vi "main.vi"() -> ()   [LabVIEW 2016]
uses:
  <vilib>/Utility/miscctls.llb/LVPointTypeDef.ctl
  <vilib>/Averna/Notify Icon/NotifyIcon.llb/BalloonIcon.ctl
  <vilib>/Averna/Notify Icon/NotifyIcon.llb/NotifyIcon.lvclass
  <vilib>/Utility/config.llb/NI_LVConfig.lvlib
  <vilib>/Utility/config.llb/Read Key (String).vi
  <vilib>/Utility/config.llb/Write Key (String).vi
  <vilib>/Utility/config.llb/Read Key (U32).vi
panel:
  in  "table元素":string
  in  "结果 2":bool
  out "数值":i32
  out "错误输出":errorcluster
  in  "连接ID":refnum<k5>
  out "结果":bool
  out "数组 2":string[](array[string])
  out "数据":string
  out "拆分包及应答Flag":string
  out "设备编码MN":string
  out "密码PW":string
  out "命令编码CN":string
  out "系统编码ST":string
  out "数组":string[](array[string])
  in  "站点名称":string(combo)
  out "时间标识":timestamp format="%<%Y/%m/%d %H:%M:%S>T"
  out "心跳包":bool
  out "空闲时间":dbl
  out "步骤":T1(ring)
  out "元素":string
  out "try":dbl
  in  "PW":string
  in  "MN":string
  in  "Port":u16
  in  "IP":string
  in  "停止 2":bool
  out "1st Error to Convert":i32(ring)=56 items=["无错误", "参数错误", "内存已满", "超出区域", "文件结束", "文件已打开", "一般文件IO错误", "未找到文件", "文件权限错误", "磁盘已满", "路径副本", "打开过多文件", "未启用", "未找到资源文件", "无法添加资源", "未找到资源", "未找到图像", "图像内存错误", "画笔不存在", "配置错误类型", "配置未找到解析段", "配置解析错误", "配置内存错误", "错误外部代码格式", "错误外部代码偏移量", "外部代码不存在", "空窗口", "销毁窗口错误", "空菜单", "打印已中止", "错误打印记录", "打印驱动程序错误", "打印时窗口错误", "打印时内存错误", "打印对话框错误", "一般打印错误", "无效设备引用句柄", "设备未找到", "设备参数错误", "设备单位错误", "无法打开设备", "设备调用已中止", "一般错误", "用户已取消", "对象ID过低", "对象ID过高", "对象不在堆中", "未知的堆", "错误DefProc ID", "DefProc不在表格中", "范围外信息", "空方法", "未知信息", "不支持管理器调用", "错误地址", "连接过程中", "连接超时", "连接过程中", "不支持网络属性", "网络错误", "正在使用的地址", "系统缺少内存", "连接已中止", "连接已拒绝", "连接未建立", "连接已建立", "连接已关闭", "初始化错误（交互应用程序管理器）", "错误事件发生", "等待无约束事件发生处理程序", "事件发生队列溢出", "错误路径", "未发出信号量", "未识别类型（交互应用程序管理器）"]
  out "读取上位机数据":string
  out "通讯包字符串":string
  out "字符串":string
  out "error out":errorcluster
  # "平台发送系统"
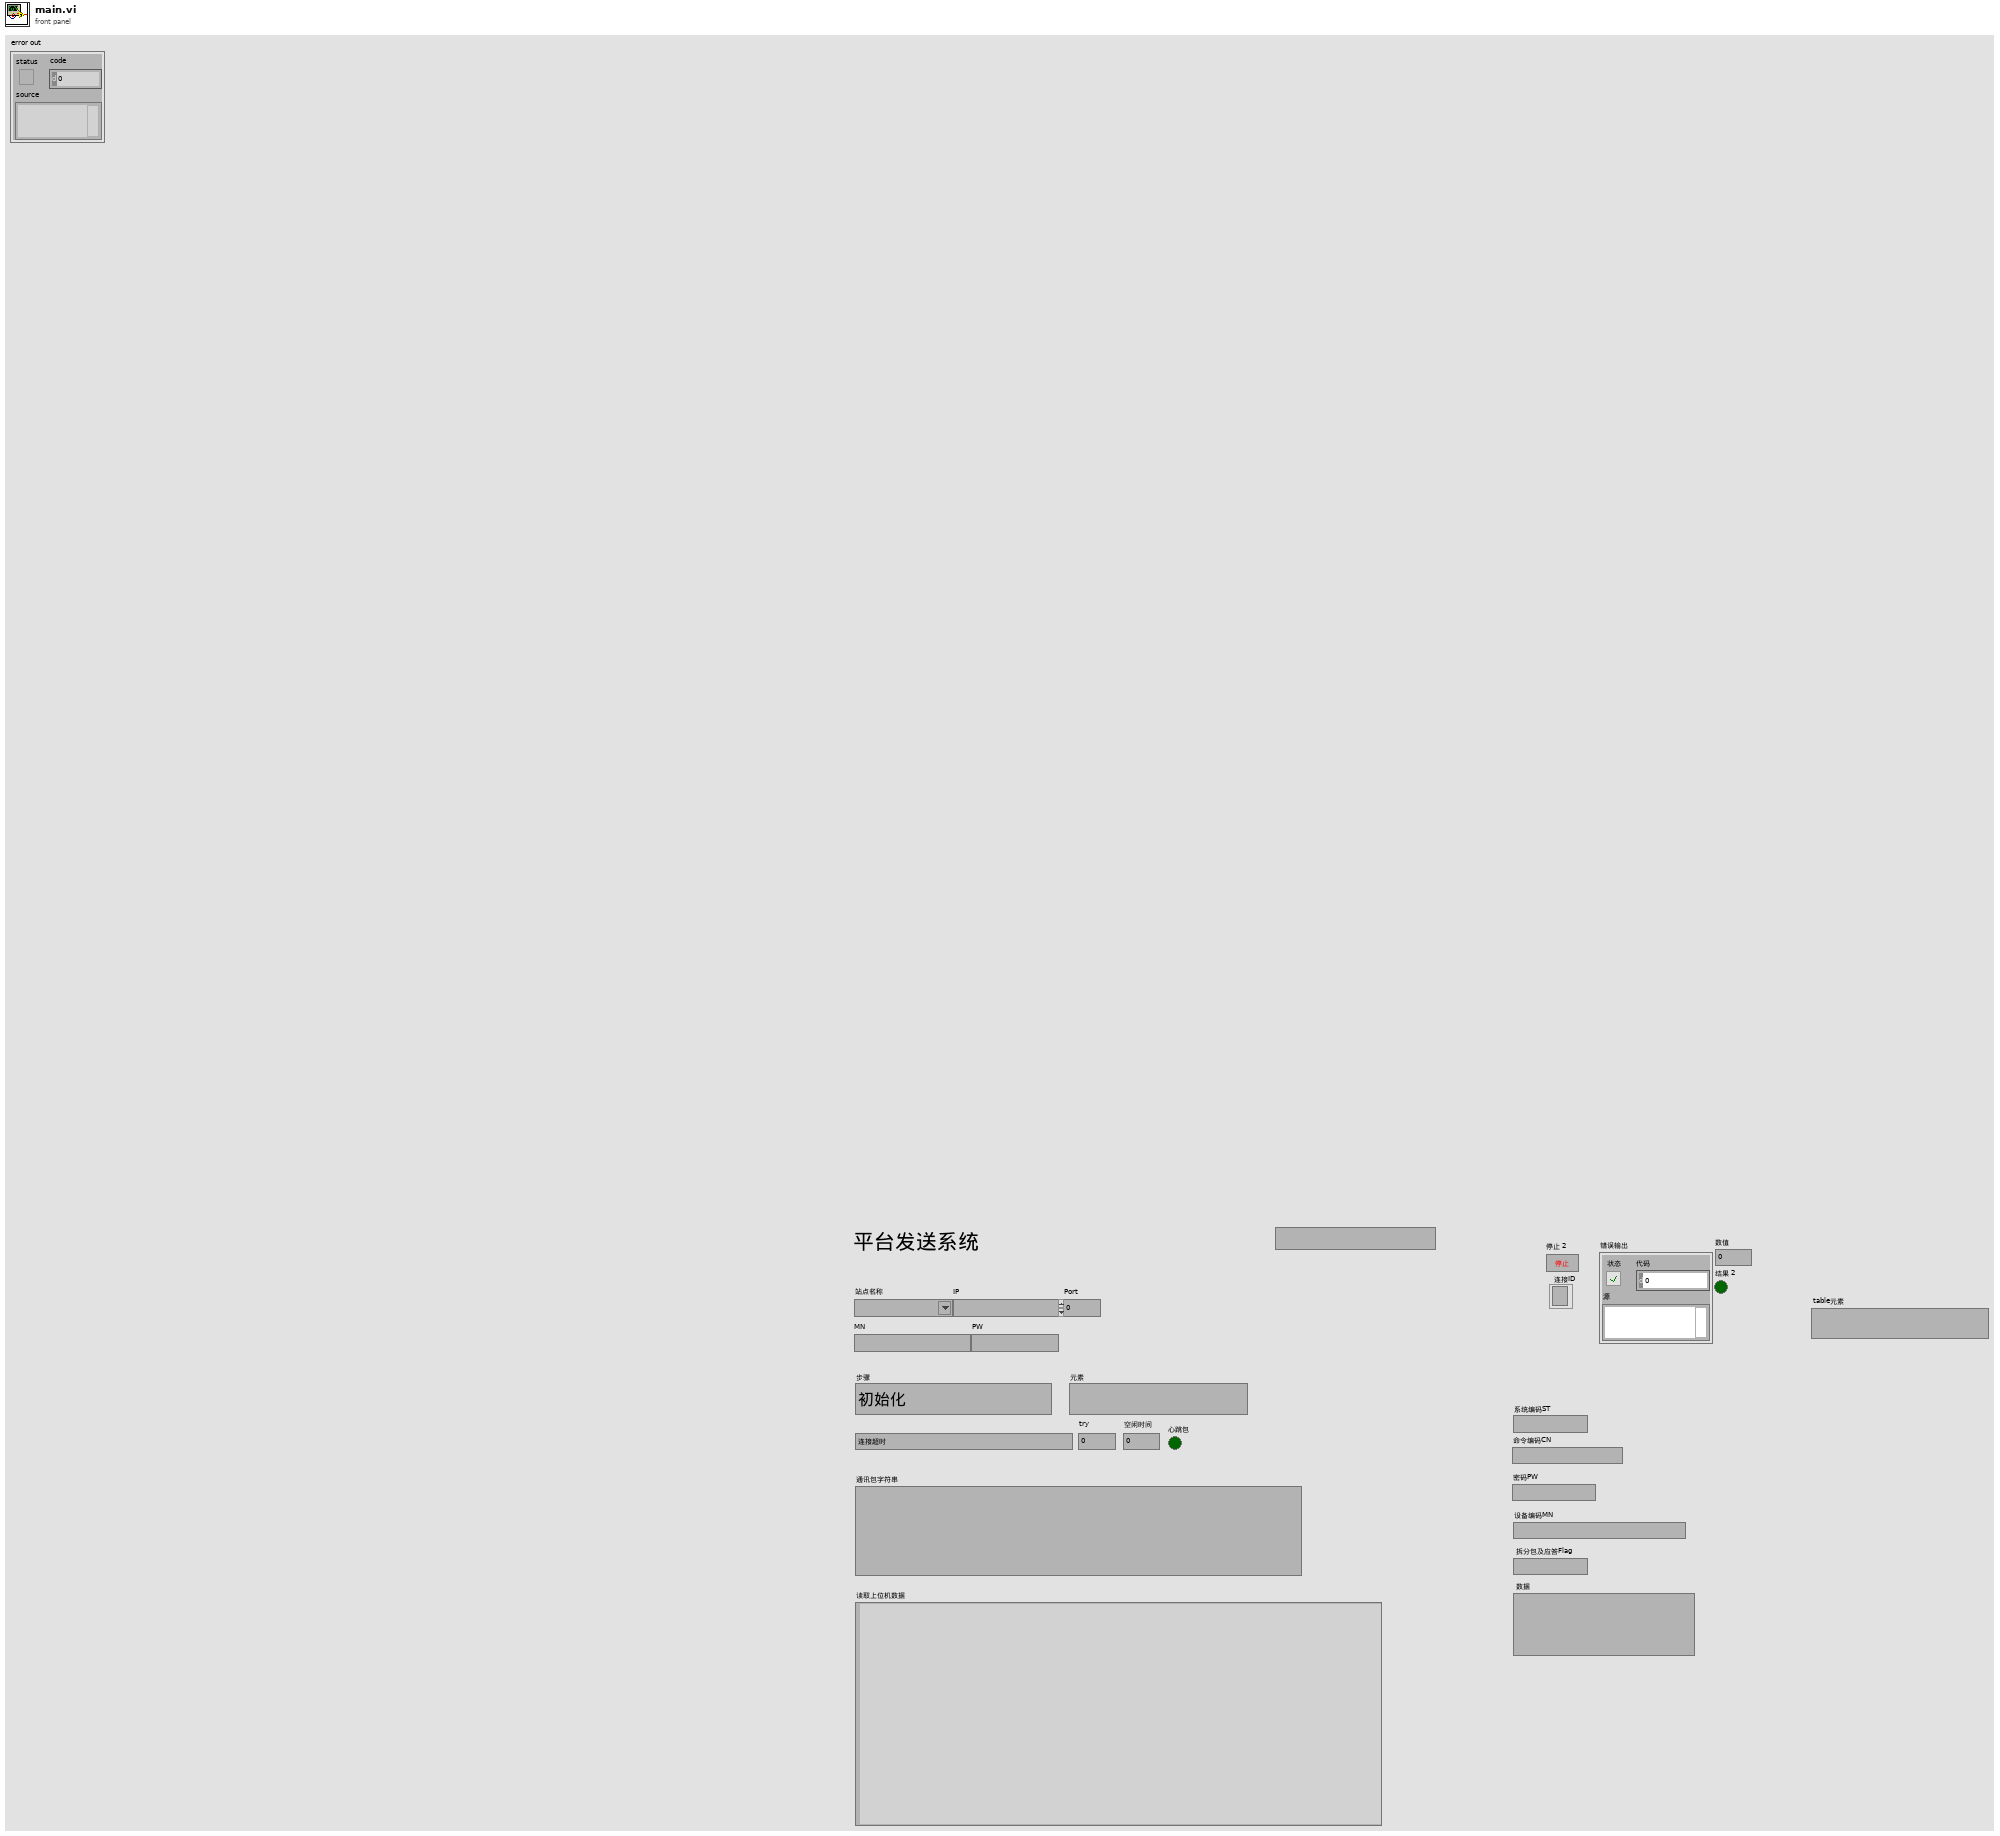
[diagram p1: front panel]
types:
  T1 = enum16{"初始化", "打开连接", "表格比对", "发送数据", "读取数据", "数据处理"}
  T2 = enum32{"invalid app kind", "Development System", "Run Time System", "Student Edition", "Embedded LabVIEW", "Evaluation", "Custom"}
  T3 = typedef "LVPointTypeDef.ctl" = cluster{"Horizontal":i16, "Vertical":i16}
  T4 = typedef "NI_LVConfig.lvlib/Config Data RefNum.ctl" = refnum<k1>
  T5 = enum32{"Bad", "Idle", "Run top level", "Running"}
  T6 = enum32{"Invalid", "Standard", "Closed", "Hidden", "Minimized", "Maximized"}
  T7 = enum16{"Standard", "Buffered", "CRLF", "Immediate"}
  T8 = typedef "NotifyIcon.lvlib/NotifyIcon.lvclass/BalloonIcon.ctl" = enum32{"None", "Information", "Warning", "Error"}
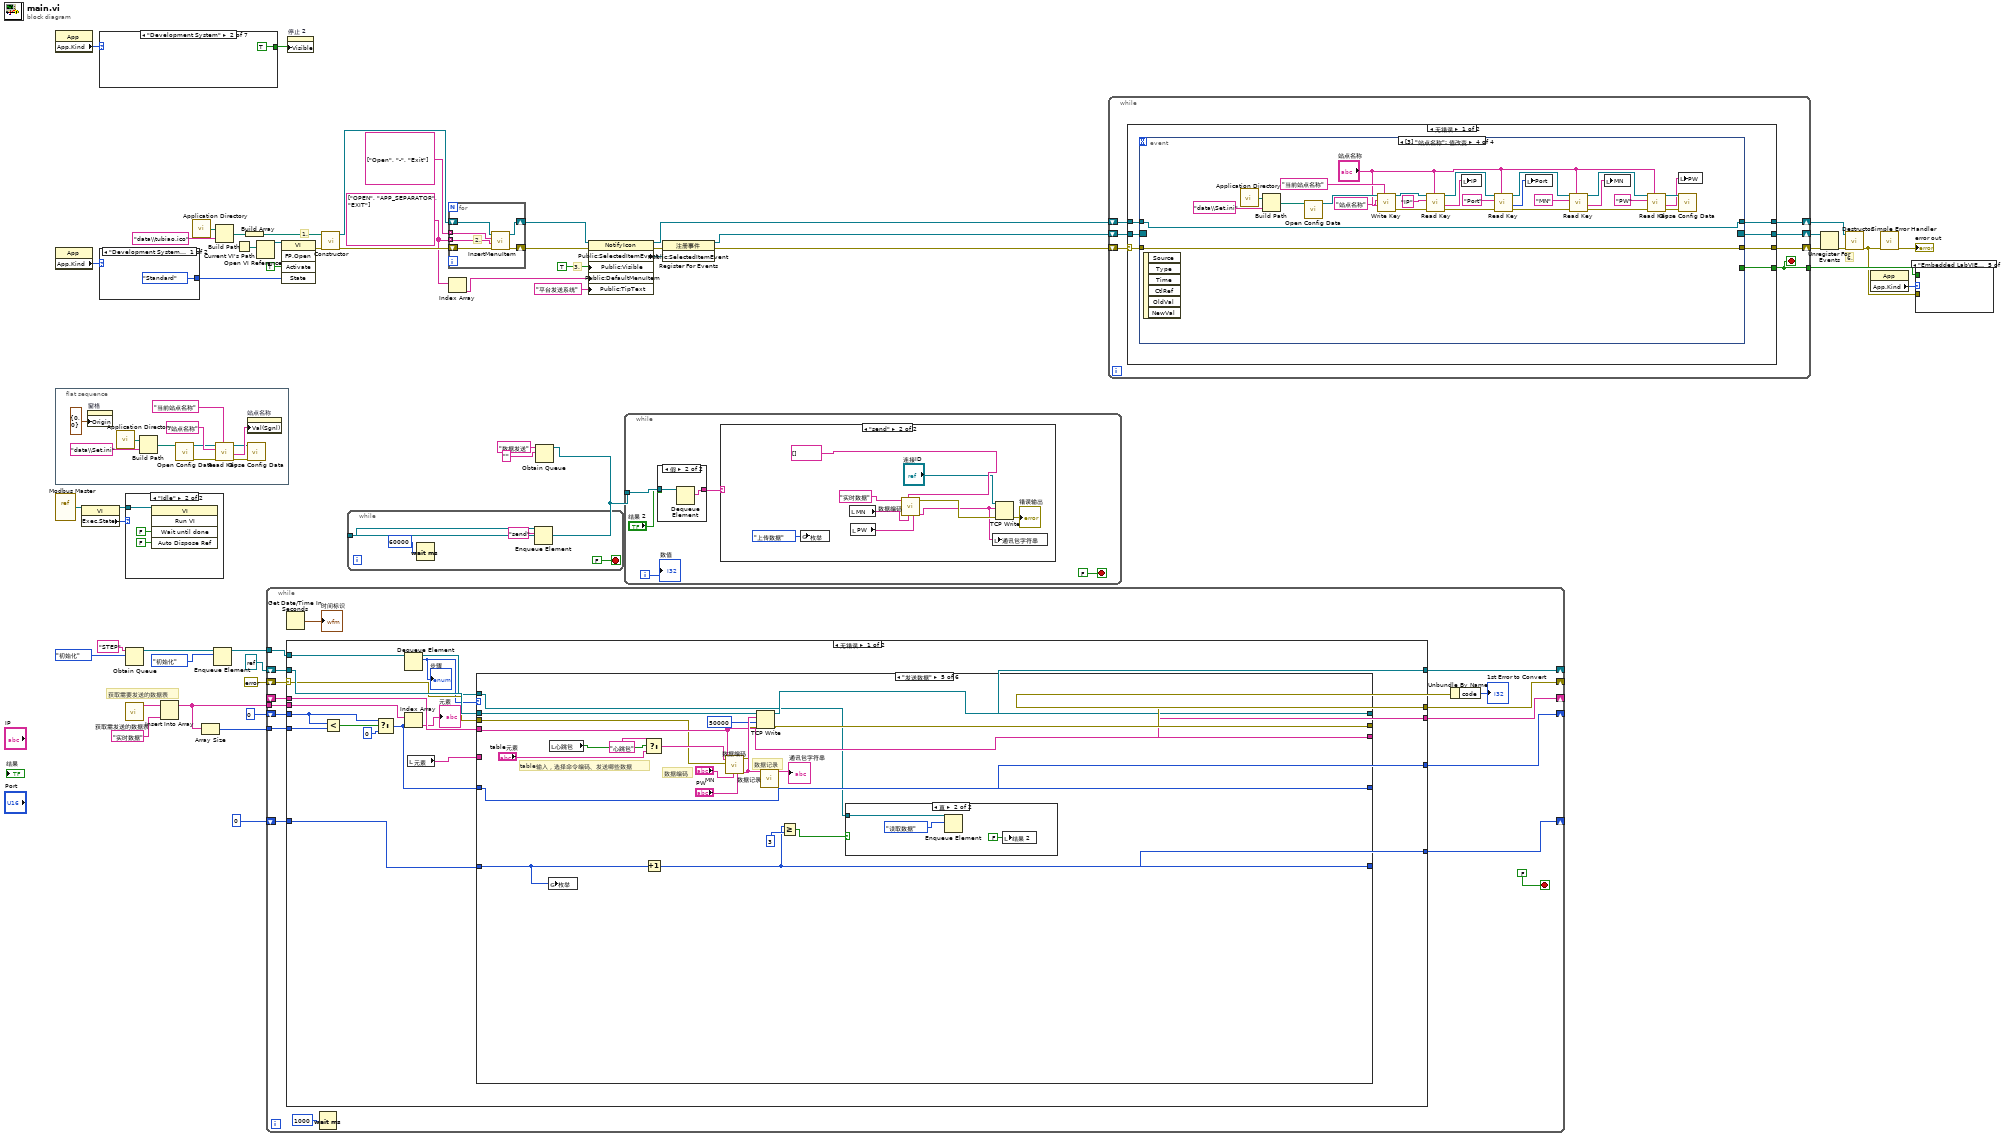
[diagram p0: block diagram]
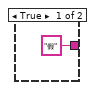
[diagram p2: hidden frame]
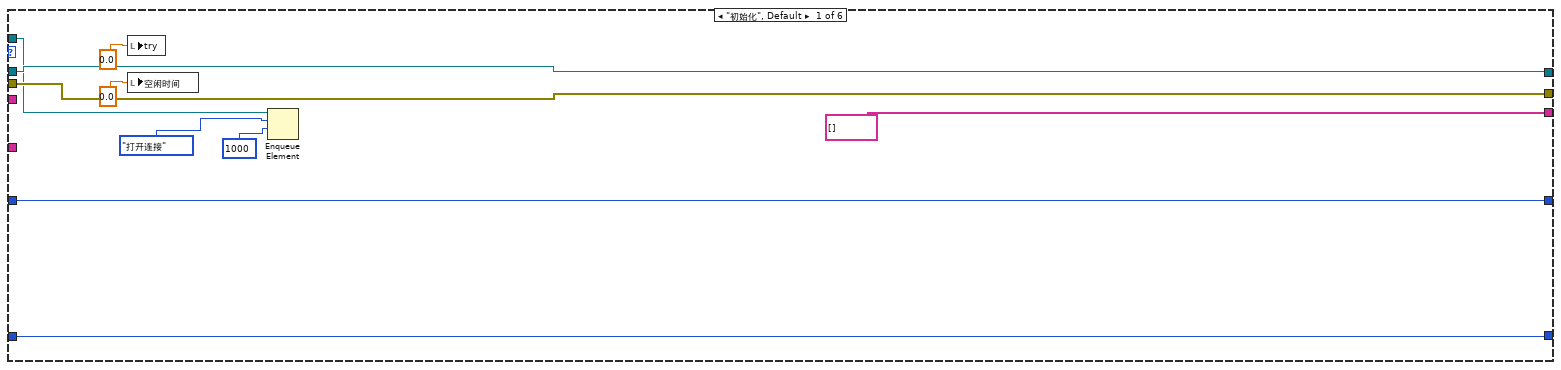
[diagram p5: hidden frame]
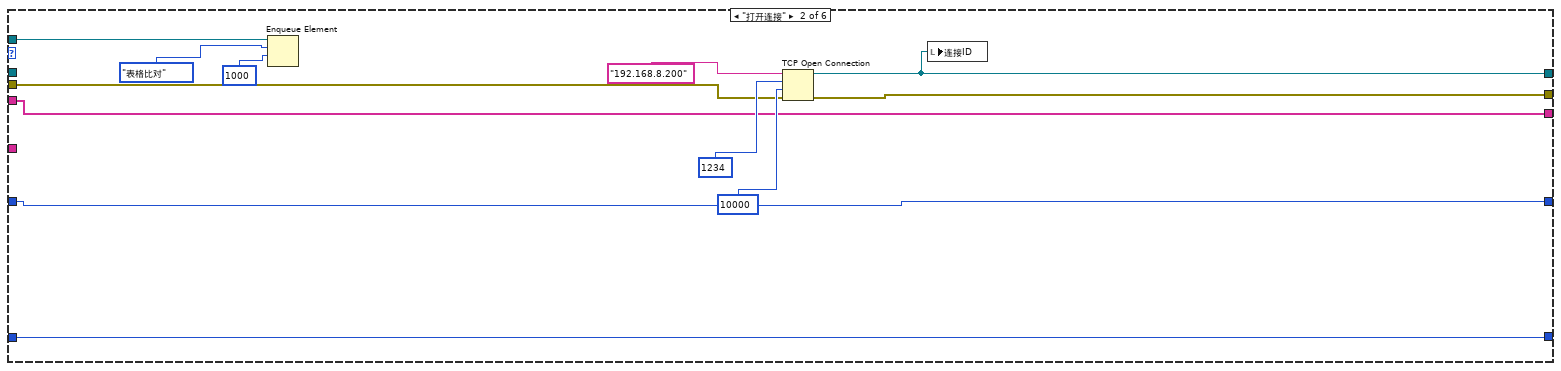
[diagram p6: hidden frame]
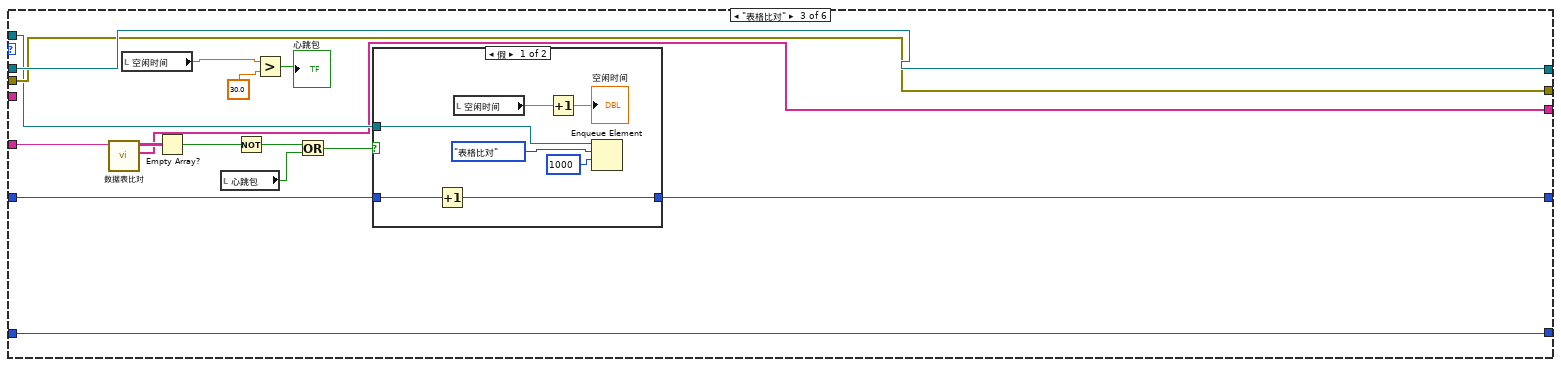
[diagram p7: hidden frame]
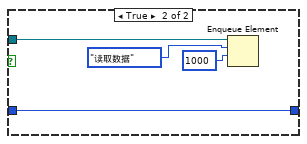
[diagram p8: hidden frame]
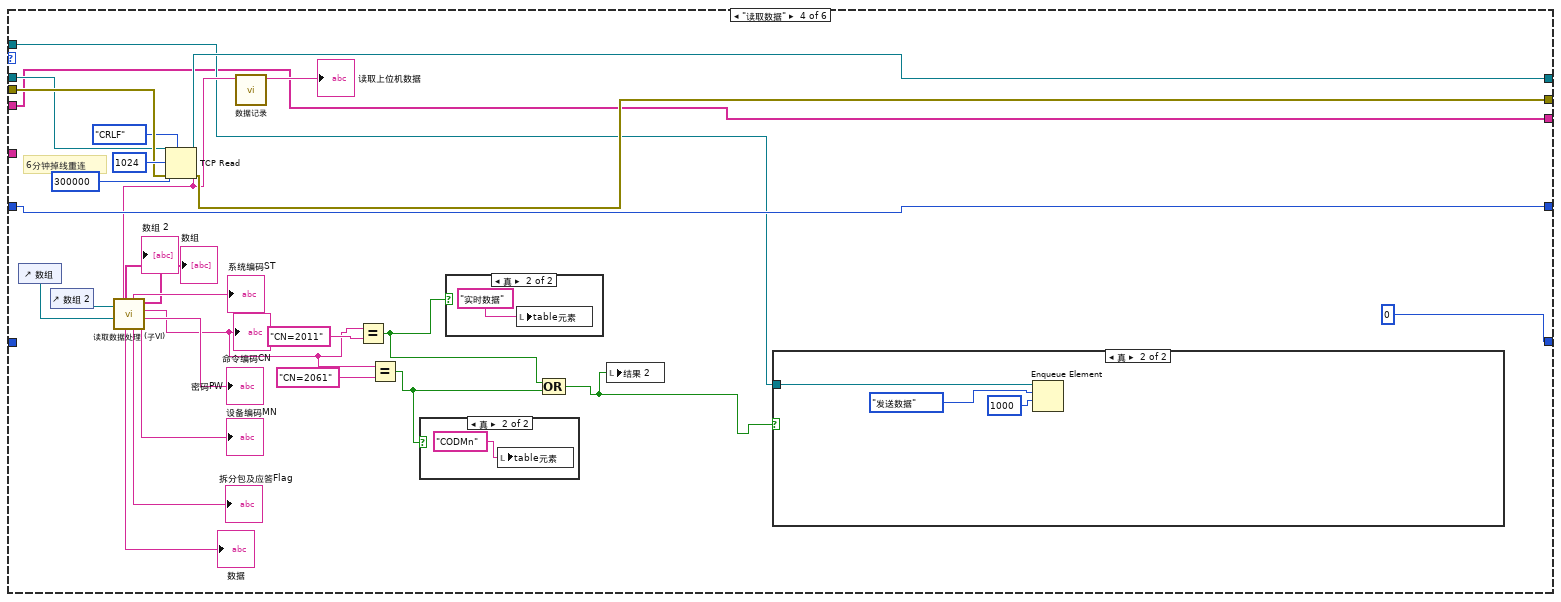
[diagram p9: hidden frame]
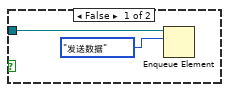
[diagram p13: hidden frame]
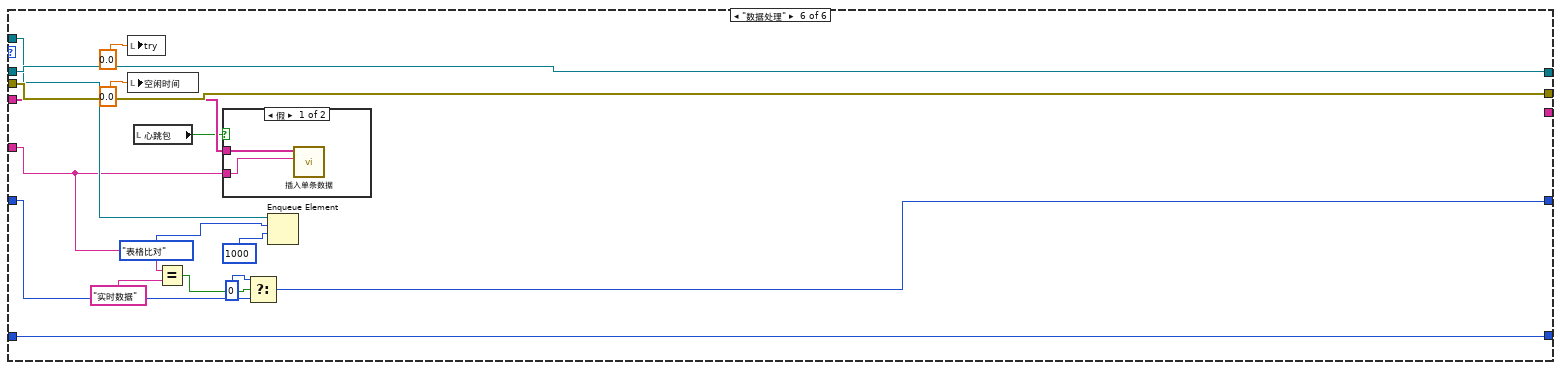
[diagram p14: hidden frame]
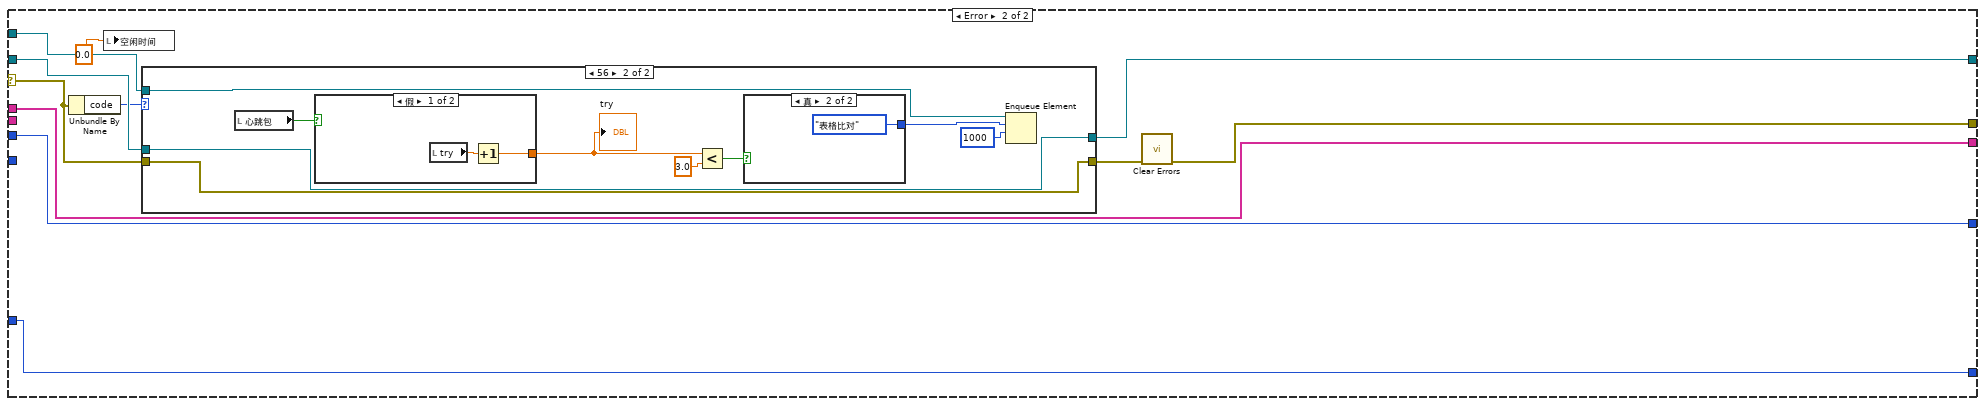
[diagram p16: hidden frame]
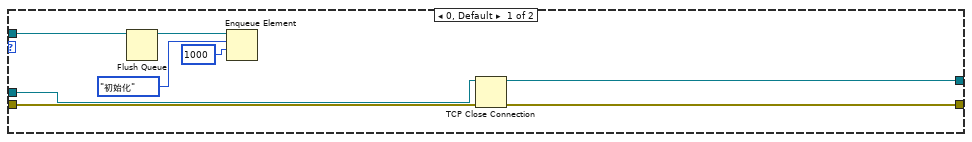
[diagram p17: hidden frame]
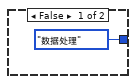
[diagram p19: hidden frame]
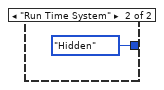
[diagram p20: hidden frame]
diagram:
  w40 = string[] ["OPEN", "APP_SEPARATOR", "EXIT"]
  # "获取需要发送的数据表"
  # "6."
  # "3."
  # "1."
  n1 = property class="App"() -> ("App.Kind"=w24:T2)  [unwired: 2 in, 2 out]
  n2 = property class="App"() -> ("App.Kind"=w21:T2)  [unwired: 2 in, 2 out]
  n3 = flat-sequence {
    frame #0 {
      n4 = property on="窗格" class="Pane"("Origin"=T3 {"Horizontal"=0, "Vertical"=0} ("原点")) -> ()  [unwired: 2 in, 2 out]
      n5 = call <vilib>:"Application Directory.vi"() -> ("Application Directory"=w56:path)
      n6 = Build Path(base path=w56, name or relative path="data\\Set.ini" ("名称或相对路径")) -> (appended path=w54:path)
      n7 = call <vilib>:"Open Config Data.vi"("configuration file path"=w54) -> ("error out"=w58:errorcluster, "refnum"=w57:T4)  [unwired: 8 in, 1 out]
      n8 = call-poly <vilib>:"Read Key.vi"("section"="当前站点名称", "error in (no error)"=w58, "key"="站点名称", "refnum"=w57) -> ("error out"=w62:errorcluster, "value"=w63:string, "refnum out"=w61:T4)  [unwired: 4 in, 1 out]
      n9 = property on="站点名称" class="CmbBox"("Val(Sgnl)"=w63) -> ()  [unwired: 2 in, 2 out]
      n10 = call <vilib>:"Close Config Data.vi"("error in (no error)"=w62, "refnum"=w61) -> ()  [unwired: 8 in, 2 out]
    }
  }
  n11 = vi-ref "Modbus Master.vi"() -> (w9:refnum<vi>)
  n12 = property class="VI"(reference=w9) -> (reference out=w7:refnum<vi>, "Exec.State"=w8:T5)  [unwired: 1 in, 1 out]
  n13 = case shown="\"Development System\"" w24 {
    tunnel: [_ TRUE ("可见") _ _ _ _ _] -> w22
    frame "invalid app kind", Default {
    }
    frame "Development System" {
    }
    frame "Run Time System" {
      n14 = call <vilib>:"Application Directory.vi"() -> ("Application Directory"=w69:path)
      n15 = Build Path(base path=w69, name or relative path="平台发送系统.exe" ("名称或相对路径")) -> (appended path=w67:path)
      n16 = call <vilib>:"FileVersionInfo.vi"("Application Path in"=w67) -> ("File Version Info"=→"字符串":string)  [unwired: 7 in, 3 out]
    }
    frame "Student Edition" {
    }
    frame "Embedded LabVIEW" {
    }
    frame "Evaluation" {
    }
    frame "Custom" {
    }
  }
  n17 = case shown="\"Development System\", 默认" w21 {
    tunnel: [T6."Standard" ("状态") T6."Hidden" ("状态")] -> w20
    frame "Development System", Default {
    }
    frame "Run Time System" {
    }
  }
  n18 = call "获取需发送的数据表.vi"() -> ("tables"=w12:string[])  [unwired: 10 in, 1 out]
  n19 = case shown="\"Idle\"" w8 {
    tunnel: w7 -> [_ w74]
    frame "Bad", Default {
    }
    frame "Idle" {
      n20 = invoke class="VI" method="Run VI"(reference=w74, "Wait until done"=FALSE ("结束前等待"), "Auto Dispose Ref"=FALSE ("自动销毁引用")) -> ()  [unwired: 2 in, 5 out]
    }
  }
  n21 = Obtain Queue(name (unnamed)="STEP" ("名称（未命名）"), element data type=T1."初始化" ("枚举")) -> (queue out=w16:refnum<queue>)  [unwired: 3 in, 2 out]
  n22 = Insert Into Array(array=w12, new element="实时数据" ("新元素/子数组")) -> (w11:string[])  [unwired: 1 in]
  n23 = call <vilib>:"Application Directory.vi"() -> ("Application Directory"=w35:path)
  n24 = Array Size(array=w11) -> (size(s)=w14:i32)
  n25 = Enqueue Element(queue=w16, element=T1."初始化" ("元素")) -> (queue out=w4:refnum<queue>)  [unwired: 2 in, 2 out]
  n26 = Build Path(base path=w35, name or relative path="data\\tubiao.ico" ("名称或相对路径")) -> (appended path=w53:path)
  n27 = Current VI's Path() -> (path=w32:path)
  n28 = Build Array(w53) -> (w43:path[])
  n29 = Open VI Reference(vi path=w32) -> (vi reference=w31:refnum<vi>)  [unwired: 5 in, 1 out]
  n30 = while {
    shift-right: [w84] -> _
    shift-left: errorcluster {"status"=FALSE, "code"=0, "source"=""} ("error out") -> [w91]
    shift-right: [w77] -> _
    shift-left: refnum<k5> refnum ("connection ID") -> [w78]
    shift-right: [w88] -> _
    shift-left: _ -> [w87]
    tunnel: w4 -> [w90]
    tunnel: w11 -> [w83]
    shift-right: [w81] -> _
    shift-left: 0 ("索引") -> [w82]
    tunnel: w14 -> [w80]
    shift-right: [w75] -> _
    shift-left: 0 ("索引") -> [w76]
    stop <- FALSE stop-if-true
    n31 = Get Date/Time In Seconds() -> (seconds since 1Jan1904=→"时间标识":timestamp)
    n32 = case shown="无错误" w91 {
      selector: w91 -> [w110 w242]
      tunnel: w78 -> [w111 w248]
      tunnel: [w105 w247] -> w77
      tunnel: [w106 w245] -> w84
      tunnel: w90 -> [w109 w240]
      tunnel: [w104 w244] -> w88
      tunnel: w87 -> [w103 w244]
      tunnel: w83 -> [w102 _]
      tunnel: w82 -> [w97 w243]
      tunnel: [w100 w243] -> w81
      tunnel: w80 -> [w99 _]
      tunnel: w76 -> [w94 w238]
      tunnel: [w93 w238] -> w75
      frame No Error {
        n33 = Less?(x=w97, y=w99) -> (x < y?=w98:bool)
        n34 = Select(t=w97, s=w98, f=0) -> (s? t:f=w96:i32)
        n35 = Dequeue Element(queue=w109) -> (queue out=w107:refnum<queue>, element=w108:T1)  [unwired: 2 in, 2 out]
        "步骤" <- w108
        n36 = Index Array(array=w102, index=w96) -> (element=→"元素":string)
        n37 = local read "元素"() -> (w92:string)
        n38 = case shown="\"发送数据\"" w108 {
          tunnel: w111 -> [w120 _ w149 w167 w214 w235]
          tunnel: w110 -> [w121 w131 w148 w187 w196 w234]
          tunnel: w107 -> [w116 w127 w146 w168 w200 w232]
          tunnel: [w121 w130 w148 w184 w203 w234] -> w106
          tunnel: [w120 w122 w149 w169 w204 w235] -> w105
          tunnel: [string[] [] ("待发送第一条数据") w129 w134 w166 w208 _] -> w104
          tunnel: w103 -> [_ w129 _ w166 w208 w233]
          tunnel: w92 -> [_ _ w144 _ _ w226]
          tunnel: w96 -> [w117 w126 w137 w185 w213 w222]
          tunnel: [w117 w126 w136 w185 w213 w223] -> w100
          tunnel: w94 -> [w112 w123 w135 _ w197 w220]
          tunnel: [w112 w123 w135 0 ("索引") w199 w220] -> w93
          frame "初始化", Default {
            n39 = local write "try"(0.0 ("try")) -> ()
            n40 = local write "空闲时间"(0.0 ("空闲时间")) -> ()
            n41 = Enqueue Element(queue=w116, element=T1."打开连接" ("元素"), timeout in ms (-1)=1000 ("超时毫秒(-1)")) -> ()  [unwired: 1 in, 3 out]
          }
          frame "打开连接" {
            n42 = Enqueue Element(queue=w127, element=T1."表格比对" ("元素"), timeout in ms (-1)=1000 ("超时毫秒(-1)")) -> ()  [unwired: 1 in, 3 out]
            n43 = TCP Open Connection(address="192.168.8.200", remote port or service name=u16 1234 ("远程端口或服务名称"), timeout ms (60000)=10000 ("超时毫秒(60000)"), error in (no error)=w131) -> (connection ID=w122:refnum<k5>, error out=w130:errorcluster)  [unwired: 1 in]
            n44 = local write "连接ID"(w122) -> ()
          }
          frame "表格比对" {
            n45 = call "数据表比对.vi"("table输入"=w144) -> ("待发送第一条数据"=w134:string[], "待发送数据"=w147:string[][])  [unwired: 8 in, 1 out]
            n46 = local read "空闲时间"() -> (w143:dbl)
            n47 = Empty Array?(array=w147) -> (empty?=w145:bool)
            n48 = local read "心跳包"() -> (w138:bool)
            n49 = Not(x=w145) -> (.not. x?=w141:bool)
            n50 = Greater?(x=w143, y=30.0) -> (0:→"心跳包":bool)
            n51 = Or(x=w141, y=w138) -> (x .or. y?=w140:bool)
            n52 = case shown="假" w140 {
              tunnel: w146 -> [w155 w160]
              tunnel: w137 -> [w151 w157]
              tunnel: [w150 w157] -> w136
              frame False {
                n53 = Increment(x=w151) -> (x+1=w150:i32)
                n54 = local read "空闲时间"() -> (w152:dbl)
                n55 = Increment(x=w152) -> (x+1=→"空闲时间":dbl)
                n56 = Enqueue Element(queue=w155, element=T1."表格比对" ("元素"), timeout in ms (-1)=1000 ("超时毫秒(-1)")) -> ()  [unwired: 1 in, 3 out]
              }
              frame True {
                n57 = Enqueue Element(queue=w160, element=T1."读取数据" ("元素"), timeout in ms (-1)=1000 ("超时毫秒(-1)")) -> ()  [unwired: 1 in, 3 out]
              }
            }
          }
          frame "读取数据" {
            # "6分钟掉线重连"
            n58 = control-ref of="数组"() -> (w181:refnum<vi>)
            n59 = control-ref of="数组 2"() -> (w180:refnum<vi>)
            n60 = TCP Read(connection ID=w167, bytes to read=1024 ("读取的字节"), error in (no error)=w187, 7:T7."CRLF" ("模式（标准）"), 9:300000 ("超时毫秒(25000)")) -> (connection ID out=w169:refnum<k5>, data out=w182:string, error out=w184:errorcluster)
            n61 = call "读取数据处理 (子VI).vi"("reference"=w181, "data out"=w182, "Array输入"=w180) -> ("设备编码MN"=→"设备编码MN":string, "密码PW"=→"密码PW":string, "命令编码CN"=w171:string, "数组 2"=→"数组 2":string[], "拆分包及应答Flag"=→"拆分包及应答Flag":string, "系统编码ST"=→"系统编码ST":string, "数据"=→"数据":string, "数组"=→"数组":string[])  [unwired: 1 in]
            "命令编码CN" <- w171
            n62 = call "数据记录.vi"("写入字段"=w182) -> ("连接的字符串"=→"读取上位机数据":string)  [unwired: 10 in]
            n63 = Equal?(x=w171, y="CN=2011") -> (x = y?=w162:bool)
            n64 = Equal?(x=w171, y="CN=2061") -> (x = y?=w161:bool)
            n65 = case shown="真" w161 {
              frame False {
              }
              frame True {
                n66 = local write "table元素"("CODMn" ("新元素/子数组")) -> ()
              }
            }
            n67 = case shown="真" w162 {
              frame False {
              }
              frame True {
                n68 = local write "table元素"("实时数据" ("新元素/子数组")) -> ()
              }
            }
            n69 = Compound Arithmetic op=OR ("复合运算")(w162, w161) -> (w164:bool)
            n70 = local write "结果 2"(w164) -> ()
            n71 = case shown="真" w164 {
              tunnel: w168 -> [_ w192]
              frame False {
              }
              frame True {
                n72 = Enqueue Element(queue=w192, element=T1."发送数据" ("元素"), timeout in ms (-1)=1000 ("超时毫秒(-1)")) -> ()  [unwired: 1 in, 3 out]
              }
            }
          }
          frame "发送数据" {
            # "table输入，选择命令编码、发送哪些数据"
            # "数据记录"
            # "数据编码"
            n73 = global write "全局1.vi" "枚举"(w197) -> ()
            n74 = local read "心跳包"() -> (w205:bool)
            n75 = Select(t="心跳包", s=w205, f="table元素") -> (s? t:f=w207:string)
            n76 = Increment(x=w197) -> (x+1=w199:i32)
            n77 = call "数据编码.vi"("PW"="PW", "MN"="MN", "CODMN"=w208, "错误常量 2"=w196, "table输入"=w207) -> ("通讯包字符串"=w211:string, "错误常量"=w198:errorcluster)  [unwired: 5 in]
            n78 = TCP Write(connection ID=w214, data in=w211, error in (no error)=w198, 9:50000 ("超时毫秒(25000)")) -> (connection ID out=w204:refnum<k5>, error out=w203:errorcluster)  [unwired: 1 out]
            n79 = call "数据记录.vi"("写入字段"=w211) -> ("连接的字符串"=→"通讯包字符串":string)  [unwired: 10 in]
            n80 = Greater Or Equal?(x=w199, y=3) -> (x >= y?=w201:bool)
            n81 = case shown="真" w201 {
              tunnel: w200 -> [w215 w218]
              frame False {
                n82 = Enqueue Element(queue=w215, element=T1."发送数据" ("元素")) -> ()  [unwired: 2 in, 3 out]
              }
              frame True {
                n83 = Enqueue Element(queue=w218, element=T1."读取数据" ("元素")) -> ()  [unwired: 2 in, 3 out]
                n84 = local write "结果 2"(FALSE ("结果 2")) -> ()
              }
            }
          }
          frame "数据处理" {
            n85 = local write "try"(0.0 ("try")) -> ()
            n86 = local write "空闲时间"(0.0 ("空闲时间")) -> ()
            n87 = local read "心跳包"() -> (w228:bool)
            n88 = Equal?(x=w226, y="实时数据") -> (x = y?=w224:bool)
            n89 = case shown="假" w228 {
              tunnel: w233 -> [w237 _]
              tunnel: w226 -> [w236 _]
              frame False {
                n90 = call "插入单条数据.vi"("table输入"=w236, "插入数据"=w237) -> ()  [unwired: 8 in, 2 out]
              }
              frame True {
              }
            }
            n91 = Select(t=0, s=w224, f=w222) -> (s? t:f=w223:i32)
            n92 = Enqueue Element(queue=w232, element=T1."表格比对" ("元素"), timeout in ms (-1)=1000 ("超时毫秒(-1)")) -> ()  [unwired: 1 in, 3 out]
          }
        }
      }
      frame Error {
        n93 = Unbundle By Name(w242) -> ("code"=w241:i32)
        n94 = local write "空闲时间"(0.0 ("空闲时间")) -> ()
        n95 = case shown="56" w241 {
          tunnel: w248 -> [w256 w265]
          tunnel: w242 -> [w255 w264]
          tunnel: [w254 w265] -> w247
          tunnel: [w253 w264] -> w246
          tunnel: w240 -> [w251 w262]
          frame 0, Default {
            n96 = Flush Queue(queue=w251) -> (queue out=w250:refnum<queue>)  [unwired: 1 in, 2 out]
            n97 = Enqueue Element(queue=w250, element=T1."初始化" ("元素"), timeout in ms (-1)=1000 ("超时毫秒(-1)")) -> ()  [unwired: 1 in, 3 out]
            n98 = TCP Close Connection(connection ID=w256, error in (no error)=w255) -> (connection ID out=w254:refnum<k5>, error out=w253:errorcluster)  [unwired: 1 in]
          }
          frame 56 {
            n99 = local read "心跳包"() -> (w258:bool)
            n100 = case shown="假" w258 {
              tunnel: [w267 _] -> w257
              frame False {
                n101 = local read "try"() -> (w266:dbl)
                n102 = Increment(x=w266) -> (x+1=w267:dbl)
              }
              frame True {
              }
            }
            "try" <- w257
            n103 = Less?(x=w257, y=3.0) -> (x < y?=w260:bool)
            n104 = case shown="真" w260 {
              tunnel: [T1."数据处理" ("枚举") T1."表格比对" ("枚举")] -> w259
              frame False {
              }
              frame True {
              }
            }
            n105 = Enqueue Element(queue=w262, element=w259, timeout in ms (-1)=1000 ("超时毫秒(-1)")) -> ()  [unwired: 1 in, 3 out]
          }
        }
        n106 = call <vilib>:"Clear Errors.vi"("error in (no error)"=w246) -> ("error out"=w245:errorcluster)  [unwired: 5 in, 1 out]
      }
    }
    n107 = Wait (ms)(milliseconds to wait=u32 1000 ("等待时间（毫秒）")) -> ()  [unwired: 1 out]
    n108 = Unbundle By Name(w84) -> ("code"=→"1st Error to Convert":i32)
  }
  n109 = invoke class="VI" method="FP.Open"(reference=w31, "Activate"=TRUE ("激活？"), "State"=w20) -> (error out=w29:errorcluster)  [unwired: 2 in, 4 out]
  n110 = property on="停止 2" class="Bool"("Visible"=w22) -> ()  [unwired: 2 in, 2 out]
  n111 = call <vilib>:"Constructor.vi"("error in"=w29, "IconFilePathList"=w43) -> ("error out"=w52:errorcluster, "NotifyIcon"=w39:refnum<class "NotifyIcon.lvclass">)  [unwired: 8 in]
  n112 = for {
    shift-right: [w274] -> w26
    shift-left: w52 -> [w275]
    tunnel: string[] ["Open", "-", "Exit"] -> [w273] mode=indexing
    tunnel: w40 -> [w272] mode=indexing
    shift-right: [w270] -> w25
    shift-left: w39 -> [w271]
    # "2."
    n113 = call <vilib>:"InsertMenuItem.vi"("error in"=w275, "ItemTag"=w272, "ItemName"=w273, "NotifyIcon in"=w271) -> ("error out"=w274:errorcluster, "NotifyIcon out"=w270:refnum<class "NotifyIcon.lvclass">)  [unwired: 6 in]
  }
  n114 = Index Array(array=w40) -> (element=w41:string)  [unwired: 1 in]
  n115 = Obtain Queue(name (unnamed)="数据发送" ("名称（未命名）"), element data type="") -> (queue out=w1:refnum<queue>)  [unwired: 3 in, 2 out]
  n116 = while {
    tunnel: w1 -> [w278]
    stop <- FALSE stop-if-true
    n117 = Wait (ms)(milliseconds to wait=u32 60000 ("等待时间（毫秒）")) -> ()  [unwired: 1 out]
    n118 = Enqueue Element(queue=w278, element="send" ("元素")) -> ()  [unwired: 2 in, 3 out]
  }
  n119 = property class="NotifyIcon"(reference=w25, error in=w26, "Public:Visible"=TRUE ("Visible"), "Public:DefaultMenuItem"=w41, "Public:TipText"="平台发送系统" ("TipText")) -> (reference out=w45:refnum<class "NotifyIcon.lvclass">, error out=w47:errorcluster, "Public:SelectedItemEvent"=w46:refnum<user-event>)
  n120 = while {
    tunnel: w1 -> [w283]
    i -> [w281]
    stop <- FALSE stop-if-true
    n121 = case shown="假" "结果 2" {
      tunnel: w283 -> [_ w287]
      tunnel: ["假" w286] -> w282
      frame True {
      }
      frame False {
        n122 = Dequeue Element(queue=w287) -> (element=w286:string)  [unwired: 2 in, 3 out]
      }
    }
    n123 = case shown="\"send\"" w282 {
      frame "假", Default {
      }
      frame "send" {
        n124 = global write "全局1.vi" "枚举"(enum16{"返回请求应答", "上传数据", "返回执行结果"}."上传数据" ("枚举")) -> ()
        n125 = local read "MN"() -> (w292:string)
        n126 = local read "PW"() -> (w293:string)
        n127 = call "数据编码.vi"("PW"=w293, "MN"=w292, "CODMN"=string[] [] ("待发送第一条数据"), "table输入"="实时数据" ("新元素/子数组")) -> ("通讯包字符串"=w294:string, "错误常量"=w296:errorcluster)  [unwired: 6 in]
        n128 = local write "通讯包字符串"(w294) -> ()
        n129 = TCP Write(connection ID="连接ID", data in=w294, error in (no error)=w296) -> (error out=→"错误输出":errorcluster)  [unwired: 1 in, 2 out]
      }
    }
    "数值" <- w281
  }
  n130 = register-events(error in=w47, w46) -> (reference out=w38:refnum<event-registration>, error out=w51:errorcluster)  [unwired: 1 in]
  n131 = while {
    shift-right: [w300] -> w49
    shift-left: w51 -> [w299]
    shift-right: [w301] -> w36
    shift-left: w45 -> [w302]
    shift-right: [w298] -> w37
    shift-left: w38 -> [w303]
    tunnel: [w297] -> w27
    stop <- w297 stop-if-true
    n132 = case shown="无错误" w299 {
      selector: w299 -> [w305 w365]
      tunnel: w303 -> [w310 w360]
      tunnel: w302 -> [w309 w361]
      tunnel: [w308 w361] -> w301
      tunnel: [w307 w363] -> w300
      tunnel: [w306 FALSE ("Discard?")] -> w297
      tunnel: [w304 w360] -> w298
      frame No Error {
        n133 = event shown="[3] \"站点名称\": 值改变" {
          selector: w310 -> [_ _ _ _]
          dyn-events: [_ _ _ _] -> w304
          timeout: _ -> [_ _ _ _]
          tunnel: w305 -> [w313 w322 w331 w359]
          tunnel: [w313 w322 w330 w359] -> w307
          tunnel: [w312 TRUE FALSE ("Discard?") _] -> w306
          tunnel: w309 -> [w311 w320 w332 w358]
          tunnel: [w311 w320 w329 w358] -> w308
          event User Event {
            # "5."
            n134 = event-data() -> ("ItemTag"=w314:string)  [unwired: 1 in]
            n135 = case shown="默认" w314 {
              tunnel: [FALSE TRUE] -> w312
              frame Default {
                n136 = Current VI's Path() -> (path=w315:path)
                n137 = Open VI Reference(vi path=w315) -> (vi reference=w316:refnum<vi>)  [unwired: 5 in, 1 out]
                n138 = invoke class="VI" method="FP.Open"(reference=w316, "Activate"=TRUE ("激活？")) -> ()  [unwired: 3 in, 5 out]
              }
              frame "EXIT" {
              }
            }
          }
          event "停止 2": Value Change {
            # "5."
            n139 = event-data() -> ()  [unwired: 1 in, 2 out]
          }
          event Panel Close? {
            # "4."
            n140 = event-data() -> ("VIRef"=w325:refnum<vi>)  [unwired: 1 in, 3 out]
            n141 = invoke class="VI" method="FP.Open"(reference=w325, "State"=T6."Hidden" ("状态")) -> ()  [unwired: 3 in, 5 out]
            n142 = call <vilib>:"ShowBalloonTip.vi"("Balloon Icon"=BalloonIcon."Information", "error in"=w331, "Text"="欢迎使用平台发送系统", "NotifyIcon in"=w332) -> ("error out"=w330:errorcluster, "NotifyIcon out"=w329:refnum<class "NotifyIcon.lvclass">)  [unwired: 6 in]
            n143 = event-data("Discard?"=TRUE ("放弃？")) -> ()  [unwired: 1 in, 1 out]
          }
          event "站点名称": Value Change {
            n144 = event-data() -> ()  [unwired: 1 in, 6 out]
            n145 = call <vilib>:"Application Directory.vi"() -> ("Application Directory"=w357:path)
            n146 = Build Path(base path=w357, name or relative path="data\\Set.ini" ("名称或相对路径")) -> (appended path=w355:path)
            n147 = call <vilib>:"Open Config Data.vi"("configuration file path"=w355) -> ("refnum"=w354:T4)  [unwired: 8 in, 2 out]
            n148 = call-poly <vilib>:"Write Key.vi"("section"="当前站点名称", "value"="站点名称", "key"="站点名称", "refnum"=w354) -> ("error out"=w341:errorcluster, "refnum out"=w353:T4)  [unwired: 5 in, 1 out]
            n149 = call-poly <vilib>:"Read Key.vi"("section"="站点名称", "error in (no error)"=w341, "key"="IP", "refnum"=w353) -> ("error out"=w340:errorcluster, "value"=w345:string, "refnum out"=w349:T4)  [unwired: 4 in, 1 out]
            n150 = local write "IP"(w345) -> ()
            n151 = call-poly <vilib>:"Read Key.vi"("section"="站点名称", "error in (no error)"=w340, "key"="Port", "refnum"=w349) -> ("error out"=w339:errorcluster, "value"=w344:u32, "refnum out"=w348:T4)  [unwired: 4 in, 1 out]
            n152 = local write "Port"(w344) -> ()
            n153 = call-poly <vilib>:"Read Key.vi"("section"="站点名称", "error in (no error)"=w339, "key"="MN", "refnum"=w348) -> ("error out"=w338:errorcluster, "value"=w343:string, "refnum out"=w347:T4)  [unwired: 4 in, 1 out]
            n154 = local write "MN"(w343) -> ()
            n155 = call-poly <vilib>:"Read Key.vi"("section"="站点名称", "error in (no error)"=w338, "key"="PW", "refnum"=w347) -> ("error out"=w337:errorcluster, "value"=w342:string, "refnum out"=w346:T4)  [unwired: 4 in, 1 out]
            n156 = local write "PW"(w342) -> ()
            n157 = call <vilib>:"Close Config Data.vi"("error in (no error)"=w337, "refnum"=w346) -> ()  [unwired: 8 in, 2 out]
          }
        }
      }
      frame Error {
        n158 = call <vilib>:"Simple Error Handler.vi"("error in (no error)"=w365) -> ("error out"=w364:errorcluster)  [unwired: 4 in, 4 out]
        n159 = call <vilib>:"Clear Errors.vi"("error in (no error)"=w364) -> ("error out"=w363:errorcluster)  [unwired: 5 in, 1 out]
      }
    }
  }
  n160 = Unregister For Events(event registration refnum=w37, error in=w49) -> (error out=w50:errorcluster)
  n161 = call <vilib>:"Destructor.vi"("error in"=w50, "NotifyIcon"=w36) -> ("error out"=w23:errorcluster)  [unwired: 9 in]
  n162 = property class="App"() -> ("App.Kind"=w28:T2)  [unwired: 2 in, 2 out]
  n163 = call <vilib>:"Simple Error Handler.vi"("error in (no error)"=w23) -> ("error out"=→"error out":errorcluster)  [unwired: 4 in, 4 out]
  n164 = case shown="\"Embedded LabVIEW\"" w28 {
    tunnel: w27 -> [_ _ w367 _ _ _ _]
    tunnel: w23 -> [_ _ _ _ _ _ _]
    frame "invalid app kind", Default {
    }
    frame "Development System" {
      n165 = Stop(stop? (T)=TRUE ("可见")) -> ()
    }
    frame "Run Time System" {
      n166 = Quit LabVIEW(quit? (T)=w367) -> ()
    }
    frame "Student Edition" {
    }
    frame "Embedded LabVIEW" {
    }
    frame "Evaluation" {
    }
    frame "Custom" {
    }
  }
